vi "Parse Empty Line.vi"(8 "error in (no error)":errorcluster, 11 "XML Refnum in":refnum<file>) -> (0 "error out":errorcluster, 3 "XML Refnum out":refnum<file>, 4 "Empty Line Found":bool)   [LabVIEW 2013, in "XML Parser.lvclass"]
uses:
  XML Parser.lvclass
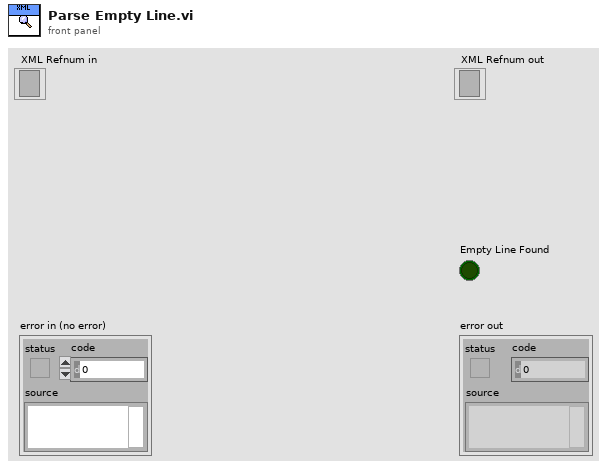
[diagram p1: front panel]
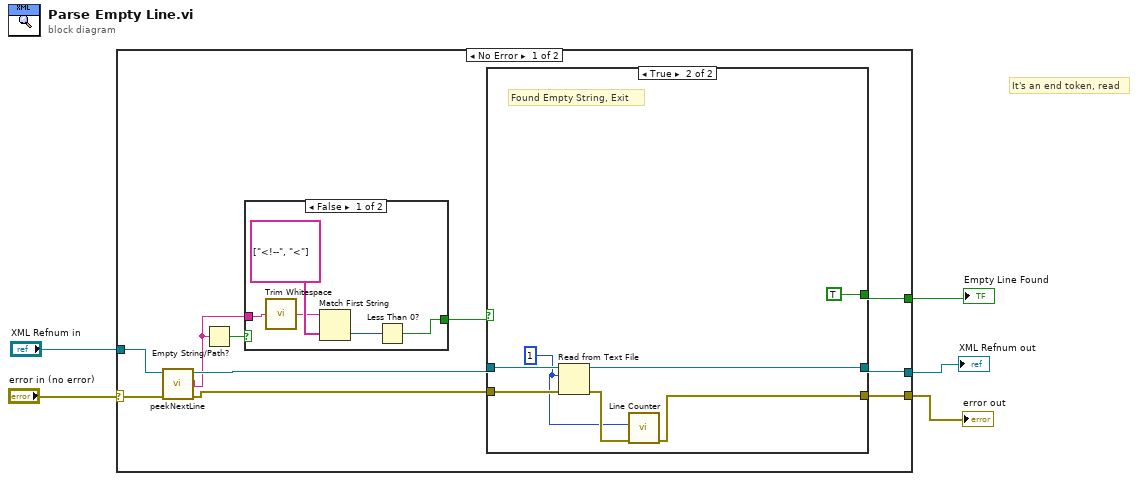
[diagram p0: block diagram]
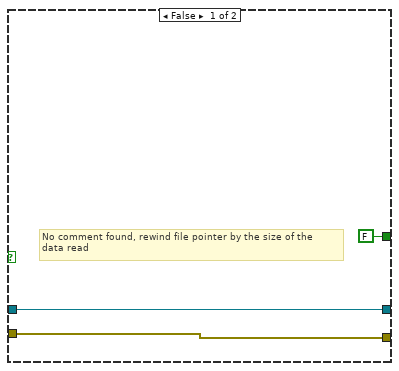
[diagram p3: hidden frame]
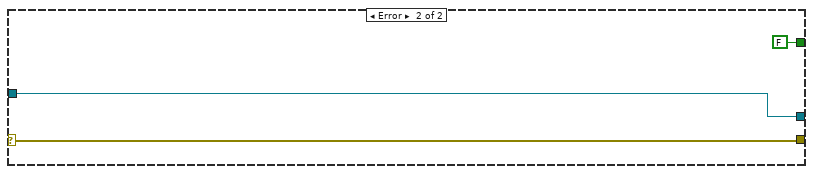
[diagram p4: hidden frame]
diagram:
  # "It's an end token, read"
  n1 = case shown="No Error" "error in (no error)" {
    selector: "error in (no error)" -> [w12 w33]
    tunnel: "XML Refnum in" -> [w11 w34]
    tunnel: [w15 w34] -> w3
    tunnel: [w14 w33] -> w2
    tunnel: [w13 FALSE] -> w1
    frame No Error {
      n2 = call "peekNextLine.vi"("error in"=w12, "file* in"=w11) -> ("error out"=w6:errorcluster, "nextLine"=w7:string, "file* out"=w10:refnum<file>)  [unwired: 7 in]
      n3 = Empty String/Path?(string/path=w7) -> (empty?=w8:bool)
      n4 = case shown="False" w8 {
        selector: w8 -> [_ w21]
        tunnel: [w18 w21] -> w9
        tunnel: w7 -> [w17 _]
        frame False {
          n5 = call <vilib>:"Trim Whitespace.vi"("string"=w17) -> ("trimmed string"=w16:string)  [unwired: 1 in]
          n6 = Match First String(2:string[] ["<!--", "<"] ("delimiters (\\s,\\t,\\r,\\n)"), 3:w16) -> (0:w20:i32)  [unwired: 1 out]
          n7 = Less Than 0?(x=w20) -> (x < 0?=w18:bool)
        }
        frame True {
        }
      }
      n8 = case shown="True" w9 {
        tunnel: w10 -> [w23 w30]
        tunnel: w6 -> [w22 w29]
        tunnel: [w23 w28] -> w15
        tunnel: [w22 w26] -> w14
        tunnel: [FALSE TRUE] -> w13
        frame False {
          # "No comment found, rewind file pointer by the size of the\ndata read"
        }
        frame True {
          w25 = 1 ("count")
          # "Found Empty String, Exit"
          n9 = Read from Text File(file (use dialog)=w30, count=w25, error in=w29) -> (refnum out=w28:refnum<file>, error out=w27:errorcluster)  [unwired: 1 in, 2 out]
          n10 = call "Line Counter.vi"("error in (no error)"=w27, "# of lines to increment (1)"=w25) -> ("error out"=w26:errorcluster)  [unwired: 8 in, 1 out]
        }
      }
    }
    frame Error {
    }
  }
  "XML Refnum out" <- w3
  "error out" <- w2
  "Empty Line Found" <- w1
